vi "fpga_Filter Constant (M Class).vi"(11 "filter delay constant":T1) -> (0 "Total Delay":u16=109, 1 "Start":fxp<+/-,4,4>=1.0, 2 "LP2 delay":u8=13, 3 "LP1 delay":u8=3, 5 "reference delay":fxp<+,22,0>)   [LabVIEW 2013, in "NI_EP_PMU_FPGA.lvlib"]
uses:
  <vilib>/addons/Electrical Power/PMU/NI_EP_PMU_FPGA.lvlib
  <vilib>/addons/Electrical Power/PMU/FPGA/subVIs/fpga_Reporting Rate Configuration.ctl
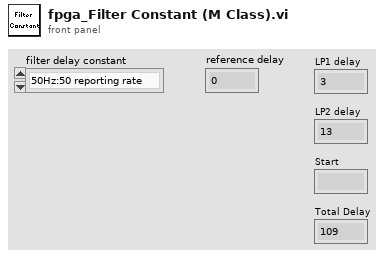
[diagram p1: front panel]
types:
  T1 = typedef "NI_EP_PMU_FPGA.lvlib/fpga_Reporting Rate Configuration.ctl" = enum16{"50Hz:50 reporting rate", "50Hz:25 reporting rate", "50Hz:10 reporting rate", "60Hz:60 reporting rate", "60Hz:30 reporting rate", "60Hz:20 reporting rate", "60Hz:15 reporting rate", "60Hz:12 reporting rate", "60Hz:10 reporting rate"}
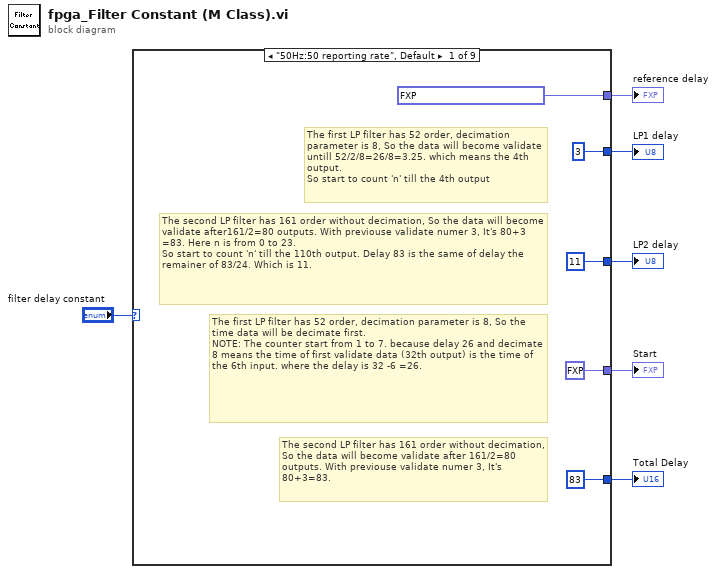
[diagram p0: block diagram]
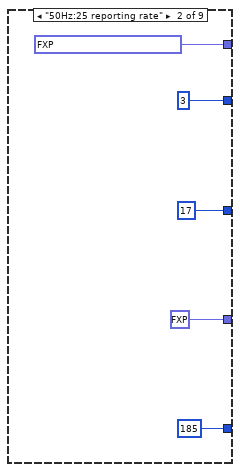
[diagram p2: hidden frame]
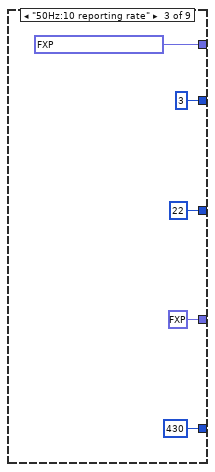
[diagram p3: hidden frame]
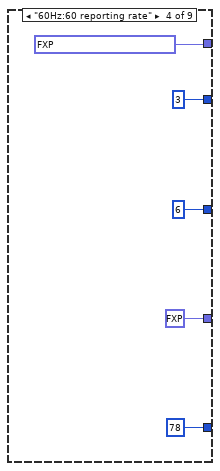
[diagram p4: hidden frame]
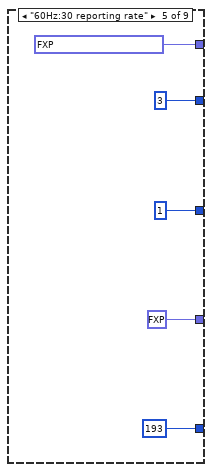
[diagram p5: hidden frame]
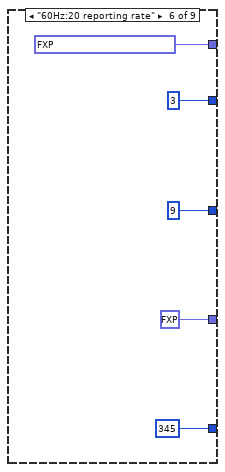
[diagram p6: hidden frame]
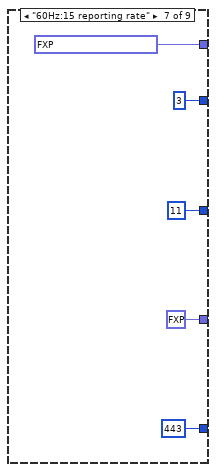
[diagram p7: hidden frame]
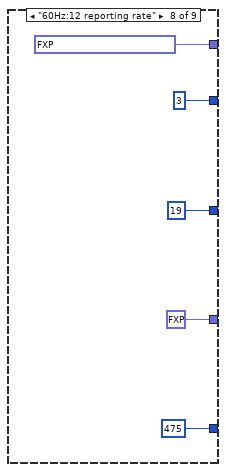
[diagram p8: hidden frame]
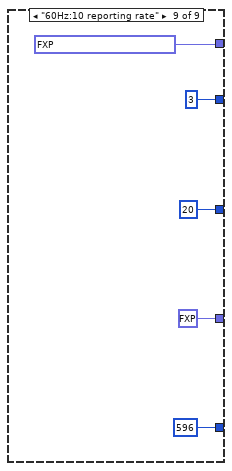
[diagram p9: hidden frame]
diagram:
  n1 = case shown="\"50Hz:50 reporting rate\", Default" "filter delay constant" {
    tunnel: [u8 3 ("n-1[0..15]") u8 3 ("n-1[0..15]") u8 3 ("n-1[0..15]") u8 3 ("n-1[0..15]") u8 3 ("n-1[0..15]") u8 3 ("n-1[0..15]") u8 3 ("n-1[0..15]") u8 3 ("n-1[0..15]") u8 3 ("n-1[0..15]")] -> w6
    tunnel: [u8 11 ("n-1[0..23]") u8 17 ("n-1[0..23]") u8 22 ("n-1[0..23]") u8 6 ("n-1[0..23]") u8 1 ("n-1[0..23]") u8 9 ("n-1[0..23]") u8 11 ("n-1[0..23]") u8 19 ("n-1[0..23]") u8 20 ("n-1[0..23]")] -> w5
    tunnel: [fxp<+/-,4,4> 1.0 ("Start") fxp<+/-,4,4> 1.0 ("Start") fxp<+/-,4,4> 1.0 ("Start") fxp<+/-,4,4> 1.0 ("Start") fxp<+/-,4,4> 1.0 ("Start") fxp<+/-,4,4> 1.0 ("Start") fxp<+/-,4,4> 1.0 ("Start") fxp<+/-,4,4> 1.0 ("Start") fxp<+/-,4,4> 1.0 ("Start")] -> w4
    tunnel: [u16 83 ("Total Delay") u16 185 ("Total Delay") u16 430 ("Total Delay") u16 78 ("Total Delay") u16 193 ("Total Delay") u16 345 ("Total Delay") u16 443 ("Total Delay") u16 475 ("Total Delay") u16 596 ("Total Delay")] -> w3
    tunnel: [fxp<+,22,0> 0.04272007942199707 ("50Hz Group Delay 4") fxp<+,22,0> 0.1217200756072998 ("50Hz Group Delay 4") fxp<+,22,0> 0.3047199249267578 ("50Hz Group Delay 4") fxp<+,21,-1> 0.04322004318237305 ("50Hz Group Delay 4") fxp<+,21,-1> 0.11721992492675781 ("50Hz Group Delay 4") fxp<+,21,-1> 0.17721986770629883 ("50Hz Group Delay 4") fxp<+,21,-1> 0.23871994018554688 ("50Hz Group Delay 4") fxp<+,21,-1> 0.298220157623291 ("50Hz Group Delay 4") fxp<+,21,-1> 0.3312201499938965 ("50Hz Group Delay 4")] -> w1
    frame "50Hz:50 reporting rate", Default {
      # "The first LP filter has 52 order, decimation parameter is 8, So the data will become validate untill 52/2/8=26/8=3.25. which means the 4th output.\nSo start to count 'n' till the 4th output"
      # "The second LP filter has 161 order without decimation, So the data will become validate after161/2=80 outputs. With previouse validate numer 3, It's 80+3 =83. Here n is from 0 to 23. \nSo start to count 'n' till the 110th output. Delay 83 is the same of delay the remainer of 83/24. Which is 11."
      # "The second LP filter has 161 order without decimation, So the data will become validate after 161/2=80 outputs. With previouse validate numer 3, It's 80+3=83."
      # "The first LP filter has 52 order, decimation parameter is 8, So the time data will be decimate first.\nNOTE: The counter start from 1 to 7. because delay 26 and decimate 8 means the time of first validate data (32th output) is the time of the 6th input. where the delay is 32 -6 =26."
    }
    frame "50Hz:25 reporting rate" {
    }
    frame "50Hz:10 reporting rate" {
    }
    frame "60Hz:60 reporting rate" {
    }
    frame "60Hz:30 reporting rate" {
    }
    frame "60Hz:20 reporting rate" {
    }
    frame "60Hz:15 reporting rate" {
    }
    frame "60Hz:12 reporting rate" {
    }
    frame "60Hz:10 reporting rate" {
    }
  }
  "Start" <- w4
  "Total Delay" <- w3
  "LP1 delay" <- w6
  "LP2 delay" <- w5
  "reference delay" <- w1
